vi "H5Sselect_none.vi"(6 "error in (no error)":errorcluster, 9 "HDF5 Space Ref":T1) -> (0 "error out":errorcluster, 3 "HDF5 Ref out":T1)   [LabVIEW 2017]
doc: "Resets the selection region to include no elements."
uses:
  <vilib>/UPVI/lvhdf5/library.llb/HDF5 Ref.ctl
  <vilib>/UPVI/lvhdf5/hdf5.dll
panel:
  # "LVHDF5 Toolkit\nCopyright (c) 2005-2013 by Jason D. Sommerville\nCopyright (c) 2014 by UPVI, LLC.\n\nThis use and distribution of this file is governed by the terms found in \nLICENSE.txt distributed with this toolkit and installed at\n <user.lib>\\_lvhdf5\\LICENSE.txt"
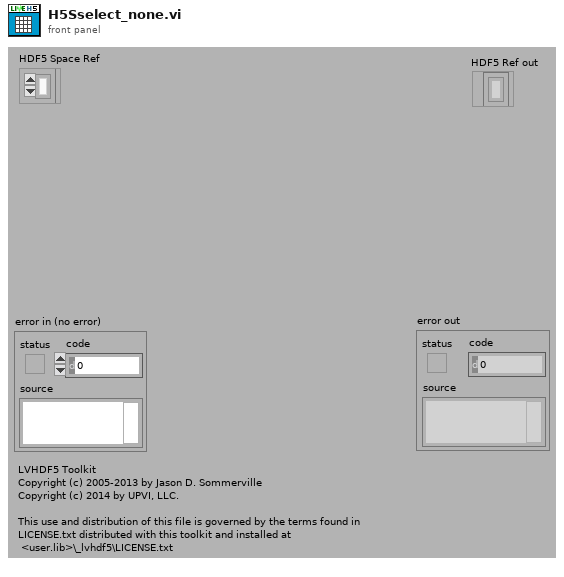
[diagram p1: front panel]
types:
  T1 = typedef "HDF5 Ref.ctl" = refnum<k1>
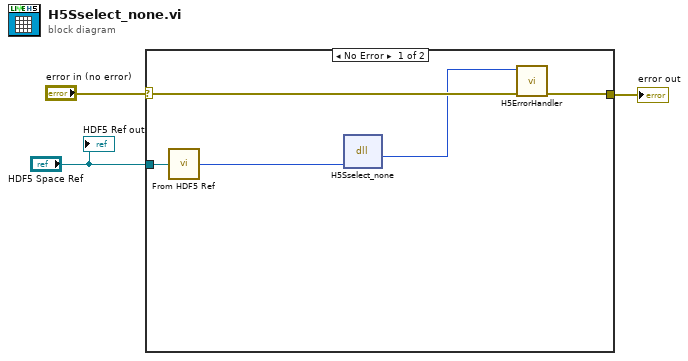
[diagram p0: block diagram]
diagram:
  n1 = case shown="No Error" "error in (no error)" {
    selector: "error in (no error)" -> [w8 w9]
    tunnel: [w7 w9] -> w2
    tunnel: "HDF5 Space Ref" -> [w6 _]
    frame No Error {
      n2 = call <vilib>:"From HDF5 Ref.vi"("HDF5 Ref"=w6) -> ("I32"=w5:i32)
      n3 = dll-call lib="C:/Program Files/National Instruments/LabVIEW 2017/vi.lib/UPVI/lvhdf5/hdf5.dll" fn="H5Sselect_none"("space_id"=w5) -> ("return type"=w4:i32)  [unwired: 4 in, 2 out]
      n4 = call <vilib>:"H5ErrorHandler.vi"("error in (no error)"=w8, "herr_t"=w4) -> ("error out"=w7:errorcluster)  [unwired: 3 in, 4 out]
    }
    frame Error {
    }
  }
  "error out" <- w2
  "HDF5 Ref out" <- "HDF5 Space Ref"
